vi "cblas zhemv.vi"(0 "A":T3, 1 "x":cdb[](array[numeric]), 2 "y":cdb[](array[numeric]), 3 "alpha":cdb=1.0+0.0i, 4 "beta":cdb=1.0+0.0i, 5 "order":T2=101 items=["CblasRowMajor"=101, "CblasColMajor"=102], 7 "uplo":T1=121 items=["CblasUpper"=121, "CblasLower"=122], 8 "lda":i32, 10 "incx":i32=1, 11 "n":i32=-1, 12 "incy":i32=1) -> (14 "zhemv":cdb[](array[numeric]), 19 "error":i32)   [LabVIEW 2020, in "NI_AALBLAS.lvlib"]
uses:
  <vilib>/Analysis/NI_AALBLAS.lvlib
  <vilib>/Analysis/Matrix/Datatypes/ComplexMatrix.ctl
  <vilib>/Analysis/BLAS.llb/Order.ctl
  <vilib>/Analysis/BLAS.llb/UpLo.ctl
  <resource>/lvblas.dll
  <vilib>/Analysis/Matrix/NI_Matrix.lvlib
panel:
  # "void cblas_zhemv(order, uplo, n, *alpha, *A, lda, *x, incx, *beta, *y, incy)"
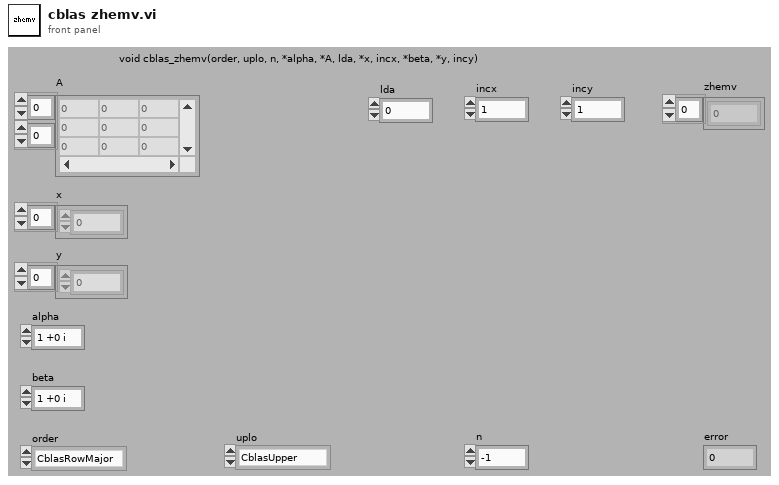
[diagram p1: front panel]
types:
  T1 = typedef "NI_AALBLAS.lvlib/UpLo.ctl" = i32
  T2 = typedef "NI_AALBLAS.lvlib/Order.ctl" = i32
  T3 = typedef "NI_Matrix.lvlib/ComplexMatrix.ctl" = cdb[][]
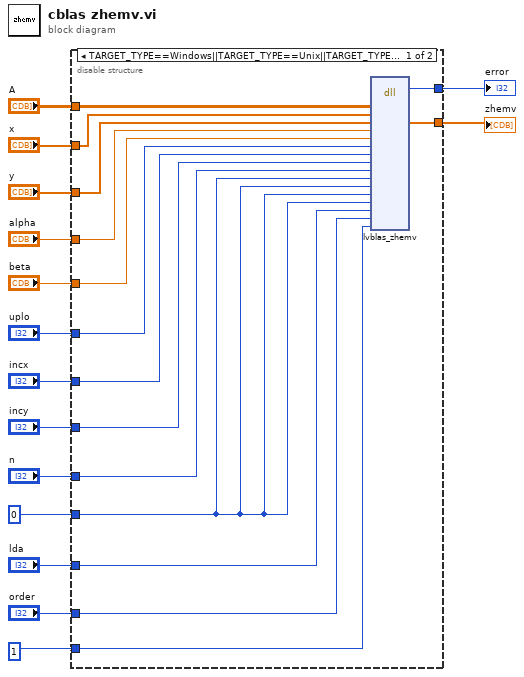
[diagram p0: block diagram]
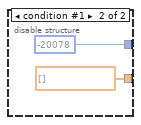
[diagram p2: hidden frame]
diagram:
  n1 = disable-structure shown="TARGET_TYPE==Windows||TARGET_TYPE==Unix||TARGET_TYPE==Mac||TARGET_TYPE==RT" {
    disable-tunnel: "x" -> [w30 _]
    disable-tunnel: "y" -> [w29 _]
    disable-tunnel: "alpha" -> [w28 _]
    disable-tunnel: [w27 cdb[] [] ("y")] -> w12
    disable-tunnel: "beta" -> [w26 _]
    disable-tunnel: "A" -> [w25 _]
    disable-tunnel: [w24 -20078 ("error")] -> w9
    disable-tunnel: 0 -> [w21 _]
    disable-tunnel: "lda" -> [w20 _]
    disable-tunnel: "uplo" -> [w23 _]
    disable-tunnel: "n" -> [w22 _]
    disable-tunnel: "order" -> [w19 _]
    disable-tunnel: "incx" -> [w18 _]
    disable-tunnel: "incy" -> [w17 _]
    disable-tunnel: 1 -> [w16 _]
    frame condition #0 (active) {
      n2 = dll-call lib="e:/builds/penguin/labview/branches/2020/dev/dist/resource/lvblas.*" fn="lvblas_zhemv" ("CBLAS.dll:MtrxxVectH")("a"=w25, "x"=w30, "y"=w29, "alpha"=w28, "beta"=w26, "uplo"=w23, "IncX"=w18, "IncY"=w17, "n"=w22, "startARow"=w21, "startACol"=w21, "startX"=w21, "startY"=w21, "lda"=w20, "order"=w19, "check"=w16) -> ("error"=w24:i32, "y"=w27:cdb[])  [unwired: 18 in, 2 out]
    }
    frame condition #1 {
    }
  }
  "zhemv" <- w12
  "error" <- w9
